vi "Opgave 6 Array sjov.vi"() -> (2 "Resultat":dbl[](array[numeric]))   [LabVIEW 2019]
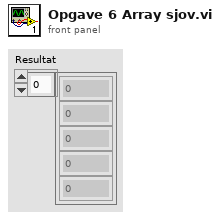
[diagram p1: front panel]
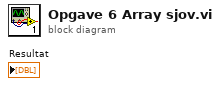
[diagram p0: block diagram]
diagram:
